vi "add filepath array.vi"(6 "priority (F)":bool, 8 "error in (no error)":errorcluster, 10 "filepath array":path[](array[path]), 11 "ComicVine_manager in":refnum<class "ComicVine_manager.lvclass">) -> (0 "error out":errorcluster, 3 "ComicVine_manager out":refnum<class "ComicVine_manager.lvclass">)   [LabVIEW 2024, in "ComicVine_manager.lvclass"]
uses:
  ComicVine_manager.lvclass
  ComicVine_manager.lvclass/ComicVine_manager.ctl
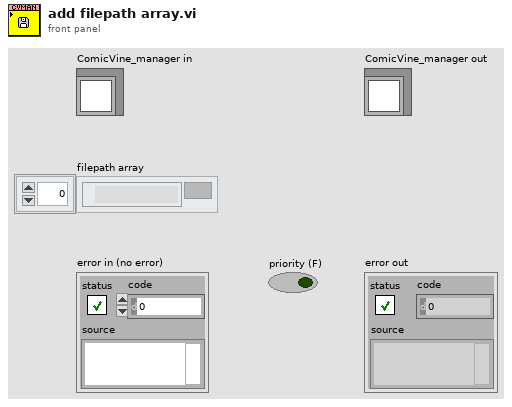
[diagram p1: front panel]
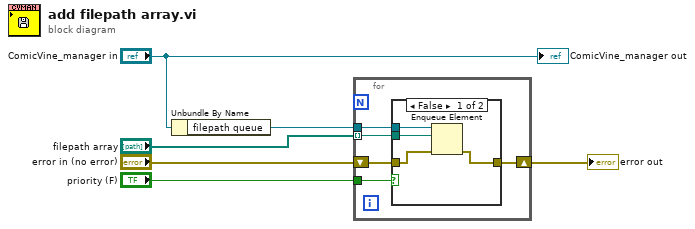
[diagram p0: block diagram]
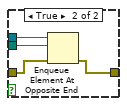
[diagram p2: hidden frame]
diagram:
  n1 = Unbundle By Name("ComicVine_manager in") -> ("filepath queue"=w6:refnum<queue>)
  n2 = for {
    tunnel: w6 -> [w11]
    tunnel: "filepath array" -> [w8] mode=indexing
    tunnel: "priority (F)" -> [w7]
    shift-right: [w9] -> w3
    shift-left: "error in (no error)" -> [w10]
    n3 = case shown="False" w7 {
      tunnel: w11 -> [w15 w19]
      tunnel: w10 -> [w14 w17]
      tunnel: [w13 w16] -> w9
      tunnel: w8 -> [w12 w18]
      frame False {
        n4 = Enqueue Element(queue=w15, element=w12, error in (no error)=w14) -> (error out=w13:errorcluster)  [unwired: 1 in, 2 out]
      }
      frame True {
        n5 = Enqueue Element At Opposite End(queue=w19, element=w18, error in (no error)=w17) -> (error out=w16:errorcluster)  [unwired: 1 in, 2 out]
      }
    }
  }
  "error out" <- w3
  "ComicVine_manager out" <- "ComicVine_manager in"
